vi "daqio_Create_Channel_Types.vi"(8 "error in (no error)":errorcluster, 10 "Channel Types":T1[](array[typedef]), 11 "daq.io type in":T2={"daq.io ref"=refnum, "daq.io API Base"="http://dashboard.daq.io/api/v1", "Device Type Key"="", "Device Key"="", "Account ID"=""}) -> (0 "error out":errorcluster, 3 "daq.io type out":T2={"daq.io ref"=refnum, "daq.io API Base"="http://dashboard.daq.io/api/v1", "Device Type Key"="", "Device Key"="", "Account ID"=""})   [LabVIEW 2013, in "daqio minimal.lvlib"]
doc: "This VI creates one or more new Channel Types for a device type. (API Route)"
uses:
  <vilib>/Easy HTTP Client/HTTP Header.ctl
  _typedefs/daqio-Type.ctl
  <vilib>/httpClient/ClientHandle.ctl
  _typedefs/daqio-Channel-Type.ctl
  daqio minimal.lvlib
  <vilib>/Easy HTTP Client/Easy HTTP.lvlib
  <vilib>/httpClient/LabVIEWHTTPClient.lvlib
panel:
  out "JSON string":string
  out "headers":T4[](array[typedef])
  out "body":string
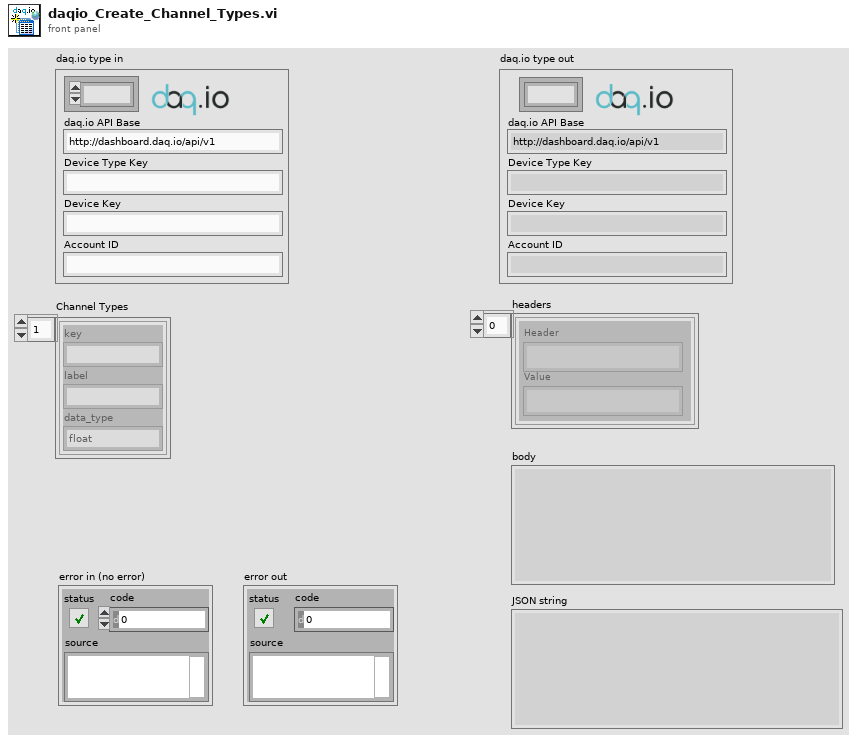
[diagram p1: front panel]
types:
  T1 = typedef "daqio minimal.lvlib/daqio-Channel-Type.ctl" = cluster{"key":string, "label":string, "data_type":string}
  T2 = typedef "daqio minimal.lvlib/daqio-Type.ctl" = cluster{"daq.io ref":T3, "daq.io API Base":string, "Device Type Key":string, "Device Key":string, "Account ID":string}
  T3 = typedef "LabVIEWHTTPClient.lvlib/ClientHandle.ctl" = refnum<k1>
  T4 = typedef "Easy HTTP.lvlib/HTTP Header.ctl" = cluster{"Header":string, "Value":string}
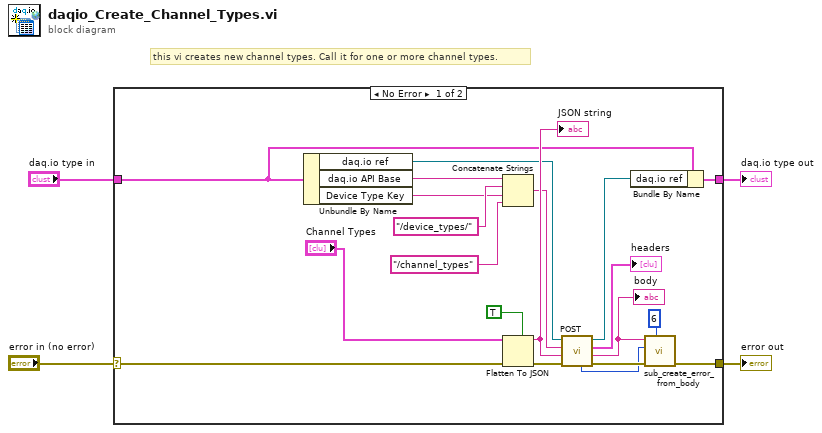
[diagram p0: block diagram]
diagram:
  # "this vi creates new channel types. Call it for one or more channel types."
  n1 = case shown="No Error" "error in (no error)" {
    selector: "error in (no error)" -> [w11 w25]
    tunnel: "daq.io type in" -> [w18 w26]
    tunnel: [w16 w26] -> w3
    tunnel: [w12 w25] -> w2
    frame No Error {
      n2 = Unbundle By Name(w18) -> ("daq.io ref"=w19:T3, "daq.io API Base"=w15:string, "Device Type Key"=w5:string)
      n3 = Concatenate Strings(w15, "/device_types/", w5, "/channel_types" ("string")) -> (w21:string)
      n4 = Flatten To JSON(enable LabVIEW extensions? (T)=TRUE, anything="Channel Types", error in (no error)=w11) -> (JSON string=w22:string, 11:w24:errorcluster)
      "JSON string" <- w22
      n5 = call <vilib>:"POST.vi"("error in (no error)"=w24, "data"=w22, "url"=w21, "client handle"=w19) -> ("error out"=w14:errorcluster, "body"=w13:string, "headers"=→"headers":T4[], "client handle out"=w17:T3, "HTTP Response Code"=w7:i32)  [unwired: 3 in]
      "body" <- w13
      n6 = Bundle By Name(cluster=w18, "daq.io ref"=w17) -> (w16:T2)
      n7 = call "sub_create_error_from_body.vi"("error code"=6, "error in (no error)"=w14, "http code"=w7, "body"=w13) -> ("error out"=w12:errorcluster)  [unwired: 7 in]
    }
    frame Error {
    }
  }
  "error out" <- w2
  "daq.io type out" <- w3
